vi "ui_override.vi"(0 "Triggering":bool, 1 "VI name":string, 5 "Parameters":bool, 7 "Stimulus":bool, 9 "Calibration":bool, 11 "error in":errorcluster, 12 "All or nothing":bool, 13 "Modes":bool) -> (4 "Override":T1, 14 "Got all":bool, 15 "error out":errorcluster)   [LabVIEW 2013]
uses:
  ui_override_opts.ctl
  ui_globals.vi
panel:
  # "String describing locker, nominally caller VI name."
  # "Which locks we got.  Pass this to update parameters."
  # "Resources that we want to control.  If the lock is available, lock it when true.  If false and we have the resource locked (as determined by \"VI name\"), then unlock."
  # "See also single_trigger_setup.vi, for the common case where we want to trigger trace cycles under program control."
  # "If true, don't lock anything unless we can get all the locks requested.  If we fail to get all the locks we will display a message box and ask whether to retry."
  # "True if we got all requested locks.  Caller should be prepared for this to be false.  If \"All or nothing\" was true, quietly aborting is reasonable, otherwise retry or some other reasonable fallback action."
  # "This VI regulates mutual exclusion on resources controlled from the user interface (micron_ui.vi).    These are primarily (but not exclusively) portions of the \"Parameters\" cluster."
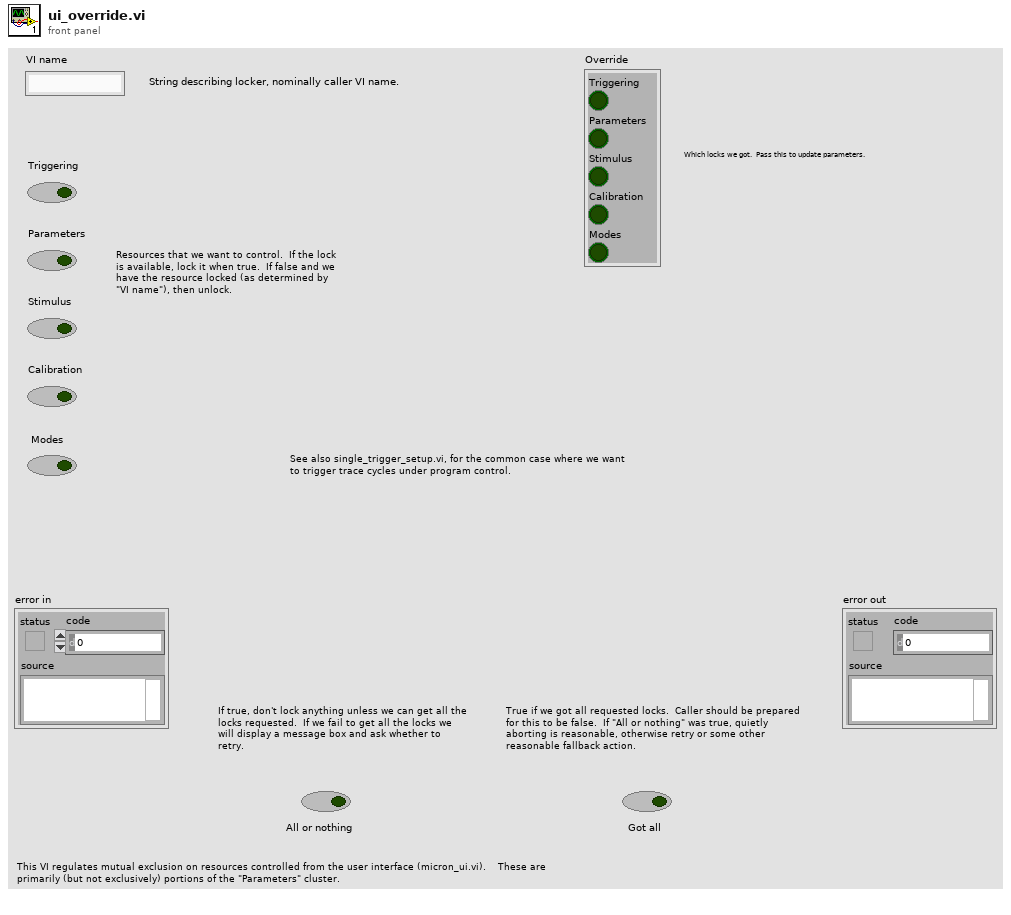
[diagram p1: front panel]
types:
  T1 = typedef "ui_override_opts.ctl" = cluster{"Triggering":bool, "Parameters":bool, "Stimulus":bool, "Calibration":bool, "Modes":bool}
  T2 = cluster{"[0]":bool, "[1]":bool, "[2]":bool, "[3]":bool, "[4]":bool}
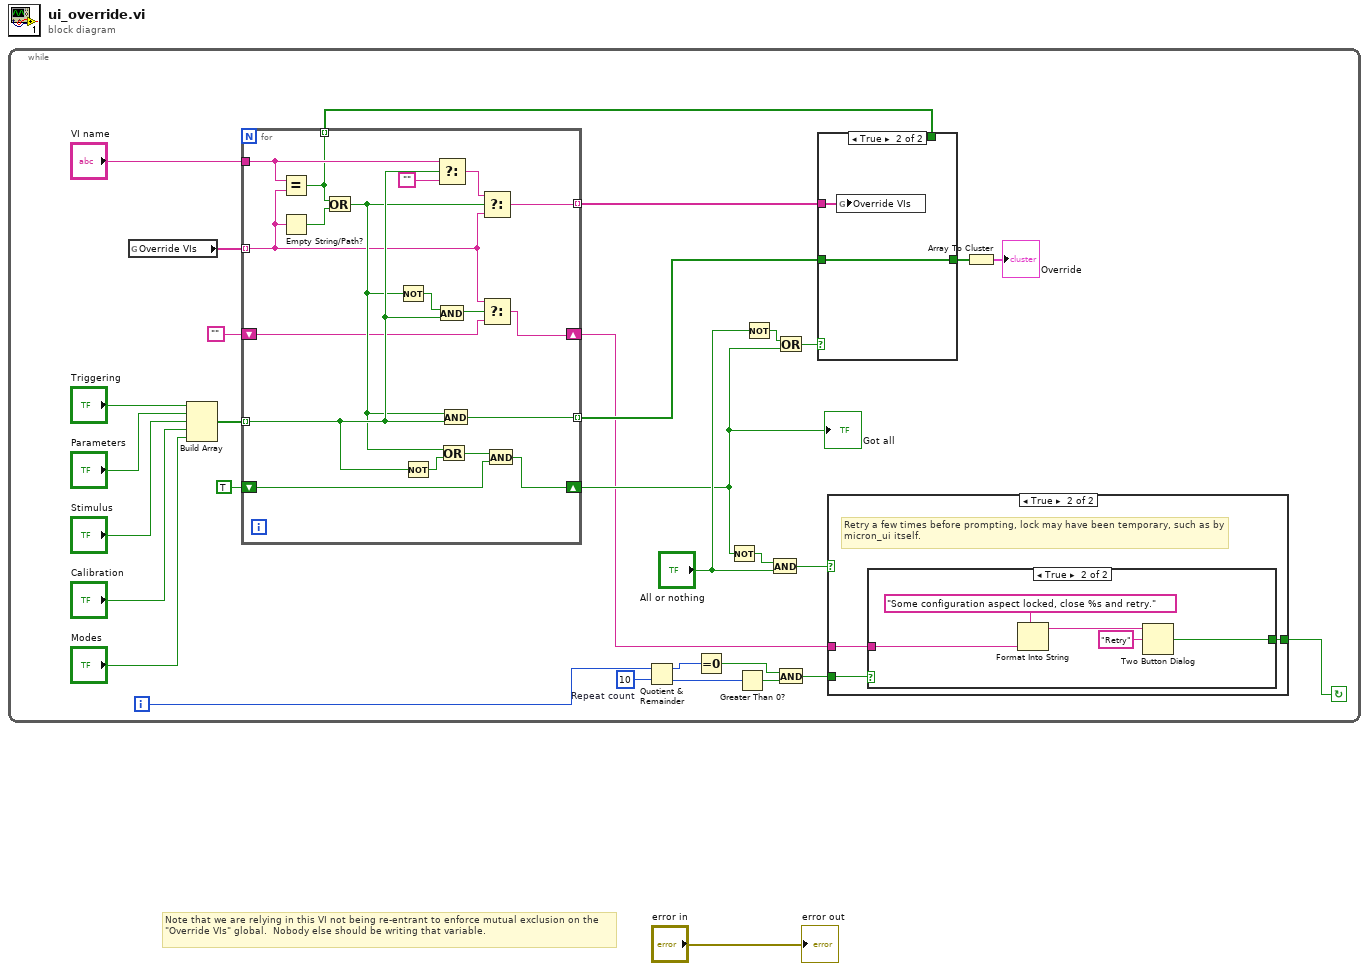
[diagram p0: block diagram]
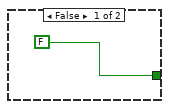
[diagram p2: hidden frame]
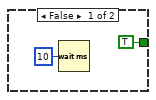
[diagram p3: hidden frame]
diagram:
  # "Note that we are relying in this VI not being re-entrant to enforce mutual exclusion on the \"Override VIs\" global.  Nobody else should be writing that variable."
  n1 = while {
    i -> [w3]
    stop <- w9 continue-if-true
    w4 = 10  # Repeat count
    n2 = global read "ui_globals.vi" "Override VIs"() -> (w25:string[])
    n3 = Build Array("Triggering", "Parameters", "Stimulus", "Calibration", "Modes") -> (w27:bool[])
    n4 = for {
      tunnel: w27 -> [w51] mode=indexing
      tunnel: "VI name" -> [w63]
      tunnel: w25 -> [w48] mode=indexing
      tunnel: [w62] -> w21 mode=indexing
      tunnel: [w61] -> w20 mode=indexing
      shift-right: [w59] -> w14
      shift-left: TRUE ("x .or. y?") -> [w60]
      tunnel: [w53] -> w17 mode=indexing
      shift-right: [w47] -> w10
      shift-left: "" -> [w46]
      n5 = Equal?(x=w63, y=w48) -> (x = y?=w53:bool)
      n6 = Empty String/Path?(string/path=w48) -> (empty?=w58:bool)
      n7 = Or(x=w53, y=w58) -> (x .or. y?=w50:bool)
      n8 = Not(x=w50) -> (.not. x?=w52:bool)
      n9 = Not(x=w51) -> (.not. x?=w56:bool)
      n10 = Select(t=w63, s=w51, f="") -> (s? t:f=w54:string)
      n11 = And(x=w52, y=w51) -> (x .and. y?=w49:bool)
      n12 = Or(x=w50, y=w56) -> (x .or. y?=w55:bool)
      n13 = And(x=w50, y=w51) -> (x .and. y?=w61:bool)
      n14 = Select(t=w54, s=w50, f=w48) -> (s? t:f=w62:string)
      n15 = Select(t=w48, s=w49, f=w46) -> (s? t:f=w47:string)
      n16 = And(x=w55, y=w60) -> (x .and. y?=w59:bool)
    }
    "Got all" <- w14
    n17 = Quotient & Remainder(x=w3, y=w4) -> (x-y*floor(x/y)=w5:i32, floor(x/y)=w6:i32)
    n18 = Equal To 0?(x=w5) -> (x = 0?=w8:bool)
    n19 = Not(x=w14) -> (.not. x?=w13:bool)
    n20 = Greater Than 0?(x=w6) -> (x > 0?=w7:bool)
    n21 = Not(x="All or nothing") -> (.not. x?=w22:bool)
    n22 = And(x=w13, y="All or nothing") -> (x .and. y?=w12:bool)
    n23 = Or(x=w22, y=w14) -> (x .or. y?=w23:bool)
    n24 = And(x=w8, y=w7) -> (x .and. y?=w2:bool)
    n25 = case shown="True" w23 {
      tunnel: w21 -> [_ w45]
      tunnel: [w43 w44] -> w19
      tunnel: w20 -> [_ w44]
      tunnel: w17 -> [w43 _]
      frame False {
      }
      frame True {
        n26 = global write "ui_globals.vi" "Override VIs"(w45) -> ()
      }
    }
    n27 = case shown="True" w12 {
      tunnel: w10 -> [_ w35]
      tunnel: [FALSE ("T button?") w34] -> w9
      tunnel: w2 -> [_ w33]
      frame False {
      }
      frame True {
        # "Retry a few times before prompting, lock may have been temporary, such as by micron_ui itself."
        n28 = case shown="True" w33 {
          tunnel: w35 -> [_ w41]
          tunnel: [TRUE ("T button?") w38] -> w34
          frame False {
            n29 = Wait (ms)(milliseconds to wait=u32 10) -> ()  [unwired: 1 out]
          }
          frame True {
            n30 = Format Into String(format string="Some configuration aspect locked, close %s and retry." ("message"), w41) -> (resulting string=w40:string)  [unwired: 2 in, 1 out]
            n31 = Two Button Dialog(message=w40, 2:"Retry" ("T button name (\"OK\")")) -> (T button?=w38:bool)  [unwired: 1 in]
          }
        }
      }
    }
    n32 = Array To Cluster(array=w19) -> (cluster=→"Override":T2)
  }
  "error out" <- "error in"
